vi "picoquant_parse_records.vi"(5 "acq_mode":T2=2 items=["T2"=2, "T3"=3], 7 "Device":T1, 8 "error in (no error)":errorcluster, 10 "overflow":u64, 11 "fifo_buffer":u32[](array[numeric])) -> (0 "error out":errorcluster, 1 "sync":u64[](array[numeric]), 2 "channels":u8[](array[numeric]), 3 "times":u64[](array[numeric]), 4 "photon_count":u64, 6 "overflow":u64)   [LabVIEW 2015]
uses:
  picoquant_Tmodes.ctl
  picoquant_devices.ctl
  lvoop_cfuncs/Debug/lvoop_cfuncs.dll
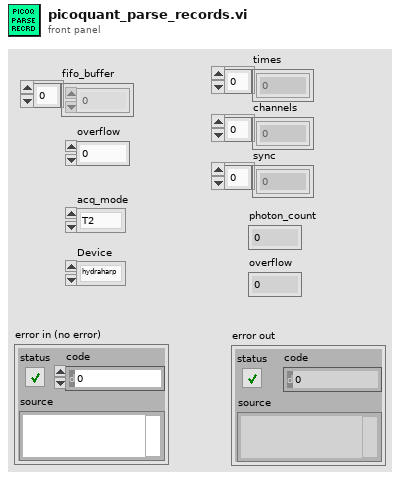
[diagram p1: front panel]
types:
  T1 = typedef "picoquant_devices.ctl" = enum16{"hydraharp", "picoharp"}
  T2 = typedef "picoquant_Tmodes.ctl" = u16
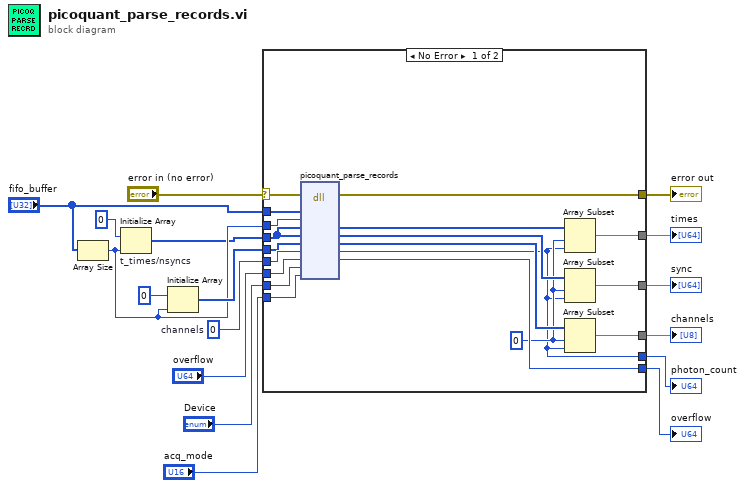
[diagram p0: block diagram]
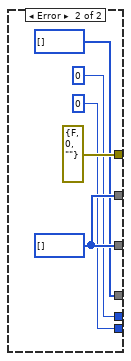
[diagram p2: hidden frame]
diagram:
  n1 = Array Size(array="fifo_buffer") -> (size(s)=w7:i32)
  n2 = Initialize Array "t_times/nsyncs"(u64 0 ("element"), w7) -> (w6:u64[])
  n3 = Initialize Array "channels"(u8 0 ("element"), w7) -> (w9:u8[])
  n4 = case shown="No Error" "error in (no error)" {
    selector: "error in (no error)" -> [w28 _]
    tunnel: [w22 w40] -> w17
    tunnel: "Device" -> [w36 _]
    tunnel: u64 0 ("overflow") -> [w35 _]
    tunnel: "acq_mode" -> [w34 _]
    tunnel: [w33 u64 0 ("overflow")] -> w13
    tunnel: [w18 u64 0 ("photon_count")] -> w12
    tunnel: [w24 w40] -> w11
    tunnel: [w20 u8[] [] ("channels")] -> w10
    tunnel: w9 -> [w32 _]
    tunnel: w7 -> [w31 _]
    tunnel: w6 -> [w30 _]
    tunnel: "fifo_buffer" -> [w29 _]
    tunnel: [w27 errorcluster {"status"=FALSE, "code"=0, "source"=""} ("error out")] -> w2
    tunnel: "overflow" -> [w26 _]
    frame No Error {
      w19 = 0 ("index")
      n5 = dll-call lib="C:/Users/bspoka/Documents/LabVIEW Data/lview_180307/lvoop_dll-master/lvoop_cfuncs/Debug/lvoop_cfuncs.dll" fn="picoquant_parse_records"(error in=w28, "fifo_buffer"=w29, "fifo_size"=w31, "macrotimes"=w30, "sync"=w30, "channels"=w32, "photon_count"=w35, "overflow"=w26, "device"=w36, "tmode"=w34) -> (error out=w27:errorcluster, "macrotimes"=w25:u64[], "sync"=w23:u64[], "channels"=w21:u8[], "photon_count"=w18:u64, "overflow"=w33:u64)  [unwired: 7 in, 1 out]
      n6 = Array Subset(array=w25, index=w19, length=w18) -> (w24:u64[])
      n7 = Array Subset(array=w23, index=w19, length=w18) -> (w22:u64[])
      n8 = Array Subset(array=w21, index=w19, length=w18) -> (w20:u8[])
    }
    frame Error {
      w40 = u64[] [] ("macrotimes")
    }
  }
  "sync" <- w17
  "overflow" <- w13
  "photon_count" <- w12
  "times" <- w11
  "channels" <- w10
  "error out" <- w2
